vi "cdex_Elevation PID.vi"(9 "elevation speed":dbl, 10 "elevation angle":dbl, 11 "elevation set point":dbl) -> (2 "Output (u)":dbl)   [LabVIEW 2015]
uses:
  <vilib>/Simulation/Implementation/Shared/SIMSCR Execution Mode.ctl
  <vilib>/Simulation/Scripting/Companion Diagram/SimConfigNode/SimParams.ctl
  <vilib>/Simulation/Scripting/Companion Diagram/SimConfigNode/_simSolvers.ctl
  <vilib>/Simulation/Param Hierarchy/Typedefs/SIMPH Param Control Actions.ctl
  <vilib>/Simulation/Implementation/Shared/SIM limit type.ctl
  <vilib>/Simulation/Implementation/Shared/NILVSim_ParamChanged.vi
  <vilib>/Simulation/Implementation/Shared/NILVSIM_BeginStep.vi
  <vilib>/Simulation/SignalArithmetic/Implementation/NILVSim Gain.llb/SIM Gain (scalar).vi
  <vilib>/Simulation/ContinuousLinear/Implementation/NILVSim Integrator new.llb/SIM Integrator distributor (scalar).vi
  <vilib>/Simulation/ContinuousLinear/Implementation/NILVSim Integrator new.llb/SIM Integrator collector (scalar).vi
  <vilib>/Simulation/Nonlinear/Implementation/NILVSim Saturation.llb/SIM Saturation (scalar).vi
  <vilib>/Simulation/Implementation/Shared/NILVSim_Manager.vi
  <vilib>/Utility/error.llb/Clear Errors.vi
  <vilib>/Simulation/Implementation/Shared/NILVSim_FinalizeModel.vi
  <vilib>/Simulation/Implementation/Shared/SIM Unbundle Sim Info.vi
  <vilib>/Simulation/Implementation/Shared/SIMSH Read Queue.vi
  3DHe_Global.vi
  <vilib>/Simulation/Implementation/Shared/NILVSim_Initialize.vi
  <vilib>/Simulation/Utility/Implementation/NILVSim Get Time and IsAcceptedStep.vi
  <vilib>/Simulation/Implementation/Shared/NILVSim_GetModelError.vi
  <vilib>/Simulation/Implementation/Shared/SIM SimErrorHandler.vi
  <vilib>/Simulation/Implementation/Shared/SIM Bundle Sim Info.vi
  <vilib>/Simulation/Scripting/Companion Diagram/SimConfigNode/SimDog.xnode
  <vilib>/Simulation/Implementation/XNodeFramework/SimXNode/SimX.xnode
  <vilib>/Simulation/ContinuousLinear/Implementation/NILVSim Integrator new.llb/SIM Integrator (scalar).vi
  <vilib>/Simulation/Implementation/Shared/NI_SIM_Implementation.lvlib
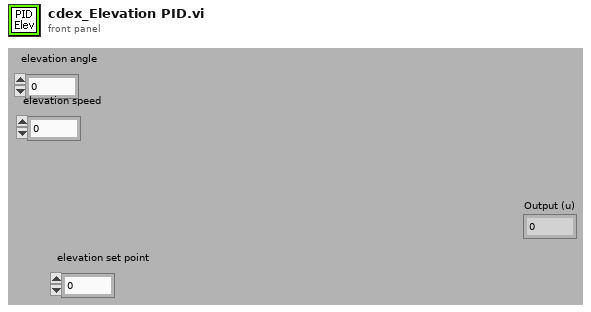
[diagram p1: front panel]
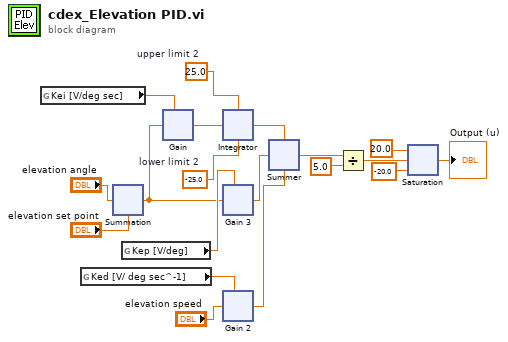
[diagram p0: block diagram]
diagram:
  w13 = -25.0  # lower limit 2
  w14 = 25.0  # upper limit 2
  n1 = global read "3DHe_Global.vi 2" "Kei [V/deg sec]"() -> (w4:dbl)
  n2 = global read "3DHe_Global.vi" "Ked [V/ deg sec^-1]"() -> (w6:dbl)
  n3 = xnode ("Summation")("Operand1"="elevation angle", "Operand2"="elevation set point") -> ("Result"=w3:dbl)
  n4 = global read "3DHe_Global.vi 3" "Kep [V/deg]"() -> (w5:dbl)
  n5 = xnode ("Gain")("gain"=w4, "input"=w3) -> ("output"=w18:dbl)  [unwired: 2 in]
  n6 = xnode ("Integrator")("upper limit"=w14, "input"=w18, "lower limit"=w13) -> ("output"=w17:dbl)  [unwired: 7 in, 2 out]
  n7 = xnode ("Gain 3")("gain"=w5, "input"=w3) -> ("output"=w19:dbl)  [unwired: 2 in]
  n8 = xnode ("Gain 2")("gain"=w6, "input"="elevation speed") -> ("output"=w15:dbl)  [unwired: 2 in]
  n9 = xnode ("Summer")("Operand1"=w17, "Operand2"=w19, "Operand3"=w15) -> ("Result"=w11:dbl)
  n10 = Divide(x=w11, y=5.0 ("Constant")) -> (x/y=w10:dbl)
  n11 = xnode ("Saturation")("upper limit"=20.0, "input"=w10, "lower limit"=-20.0) -> ("output"=→"Output (u)":dbl)  [unwired: 2 in]
